vi "datatocsv.vi"(10 "FIT RESULTS":T1(array[cluster]), 11 "fit result data":cluster{"all rows":dbl[], "all rows":dbl[]}[](array[cluster])) -> (3 "error out":errorcluster)   [LabVIEW 2020]
uses:
  <vilib>/Utility/sysdir.llb/System Directory Type.ctl
panel:
  out "peakdata":string
  out "pltot data string":string
  out "path":path
  out "Array":dbl[][](array[numeric])
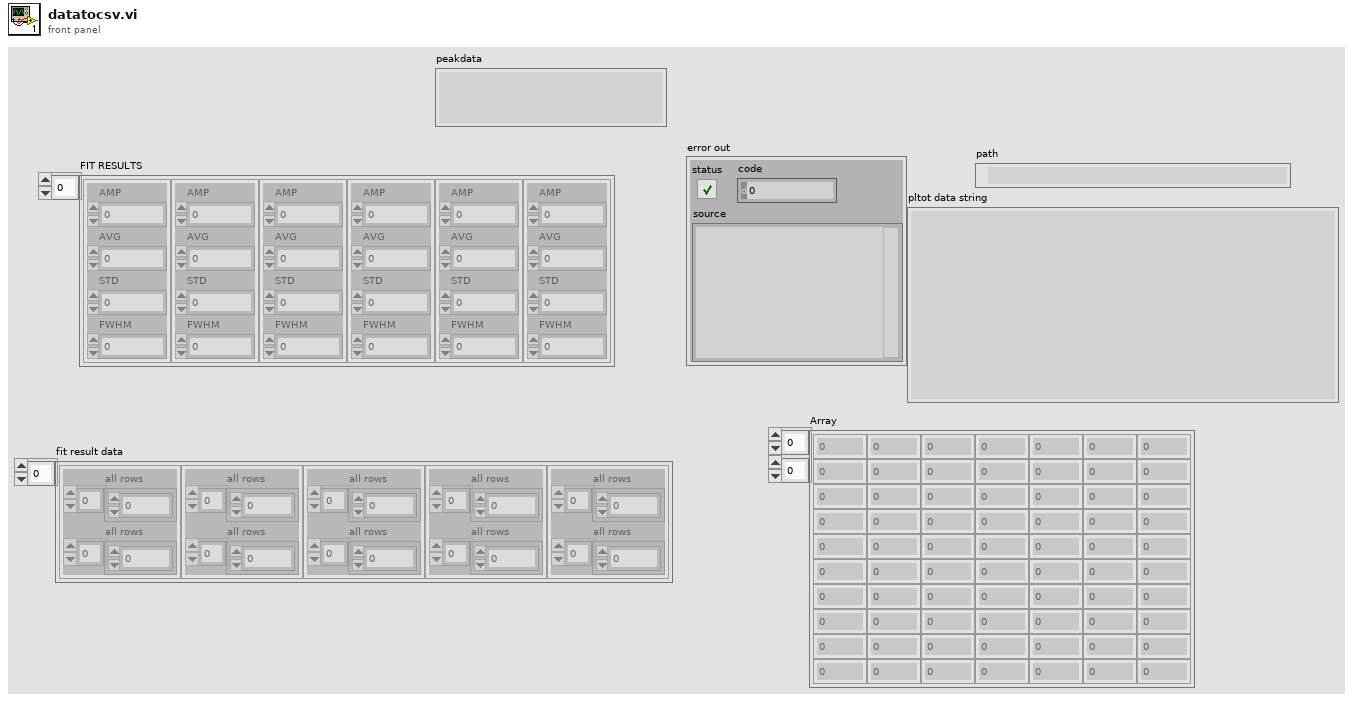
[diagram p1: front panel]
types:
  T1 = cluster{"AMP":dbl, "AVG":dbl, "STD":dbl, "FWHM":dbl}[]
  T2 = enum16{"open", "replace", "create", "open or create", "replace or create", "replace or create with confirmation"}
  T3 = typedef "System Directory Type.ctl" = i32
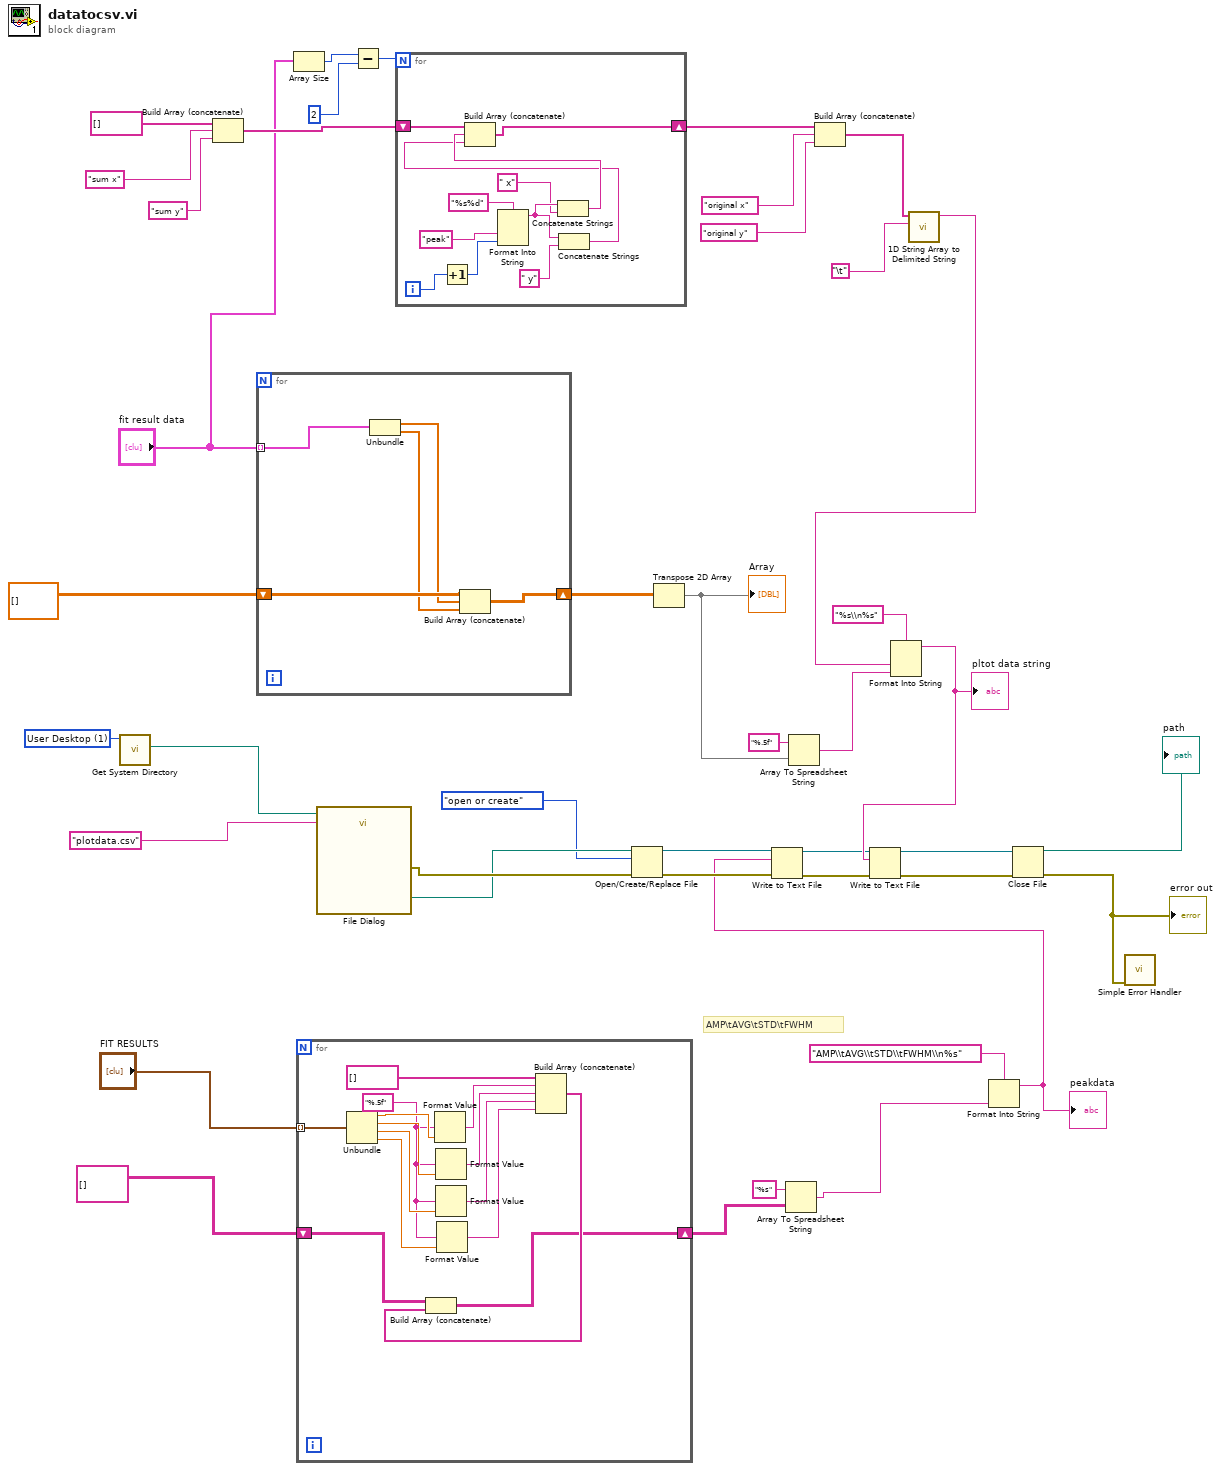
[diagram p0: block diagram]
diagram:
  w16 = T3 1 items=["User Home"=0, "User Desktop"=1, "User Documents"=2, "User Application Data"=3, "User Preferences"=4, "User Temporary"=5, "Public Documents"=6, "Public Application Data"=7, "Public Preferences"=8, "Public Cache"=13, "System Core Libraries"=9, "System Installed Libraries"=10, "Application Files"=11, "Boot Volume Root"=12] ("system directory type")
  # "AMP\\tAVG\\tSTD\\tFWHM"
  n1 = call <vilib>:"Get System Directory.vi"("system directory type"=w16) -> ("system directory"=w7:path)  [unwired: 10 in]
  n2 = Build Array (concatenate)(string[] [], "sum x", "sum y" ("element")) -> (w28:string[])
  n3 = for {
    tunnel: "fit result data" -> [w47] mode=indexing
    shift-right: [w43] -> w35
    shift-left: dbl[][] [] -> [w46]
    n4 = Unbundle(w47) -> ("all rows"=w45:dbl[], "all rows"=w44:dbl[])
    n5 = Build Array (concatenate)(w46, w45, w44) -> (w43:dbl[][])
  }
  n6 = Array Size(array="fit result data") -> (size(s)=w9:i32)
  n7 = for {
    tunnel: "FIT RESULTS" -> [w60] mode=indexing
    shift-right: [w57] -> w40
    shift-left: string[][] [] -> [w61]
    w48 = "%.5f" ("format string")
    n8 = Unbundle(w60) -> ("AMP"=w56:dbl, "AVG"=w55:dbl, "STD"=w54:dbl, "FWHM"=w53:dbl)
    n9 = Format Value(format string=w48, value (0)=w56) -> (output string=w52:string)  [unwired: 1 in]
    n10 = Format Value(format string=w48, value (0)=w55) -> (output string=w51:string)  [unwired: 1 in]
    n11 = Format Value(format string=w48, value (0)=w54) -> (output string=w50:string)  [unwired: 1 in]
    n12 = Format Value(format string=w48, value (0)=w53) -> (output string=w49:string)  [unwired: 1 in]
    n13 = Build Array (concatenate)(string[] [], w52, w51, w50, w49) -> (w58:string[])
    n14 = Build Array (concatenate)(w61, w58) -> (w57:string[][])
  }
  n15 = call "File Dialog"("start path"=w7, "default name"="plotdata.csv") -> ("selected path"=w12:path, "error out"=w17:errorcluster)  [unwired: 10 in, 2 out]
  n16 = Subtract(x=w9, y=2) -> (x-y=w27:i32)
  n17 = for {
    N: w27 -> [_]
    shift-right: [w67] -> w26
    shift-left: w28 -> [w71]
    i -> [w72]
    n18 = Increment(x=w72) -> (x+1=w68:i32)
    n19 = Format Into String(format string="%s%d", "peak", w68) -> (resulting string=w66:string)  [unwired: 2 in, 1 out]
    n20 = Concatenate Strings(w66, " x" ("string")) -> (w63:string)
    n21 = Concatenate Strings(w66, " y" ("string")) -> (w62:string)
    n22 = Build Array (concatenate)(w71, w63, w62) -> (w67:string[])
  }
  n23 = Open/Create/Replace File(file path (use dialog)=w12, error in=w17, operation (0:open)=T2."open or create") -> (refnum out=w5:refnum<file>, error out=w4:errorcluster)  [unwired: 3 in, 1 out]
  n24 = Transpose 2D Array(2D array=w35) -> (transposed array=w34:dbl[][])
  "Array" <- w34
  n25 = Array To Spreadsheet String(array=w40, 3:"%s" ("format string")) -> (spreadsheet string=w37:string)  [unwired: 1 in]
  n26 = Array To Spreadsheet String(array=w34, 3:"%.5f" ("format string")) -> (spreadsheet string=w32:string)  [unwired: 1 in]
  n27 = Build Array (concatenate)(w26, "original x", "original y") -> (w22:string[])
  n28 = call <vilib>:"1D String Array to Delimited String.vi"("delimiter"="\t", "string array"=w22) -> ("delimited string"=w20:string)  [unwired: 9 in]
  n29 = Format Into String(format string="%s\\n%s", w20, w32) -> (resulting string=w6:string)  [unwired: 2 in, 1 out]
  "pltot data string" <- w6
  n30 = Format Into String(format string="AMP\\tAVG\\tSTD\\tFWHM\\n%s", w37) -> (resulting string=w1:string)  [unwired: 2 in, 1 out]
  "peakdata" <- w1
  n31 = Write to Text File(file (use dialog)=w5, text=w1, error in=w4) -> (refnum out=w3:refnum<file>, error out=w2:errorcluster)  [unwired: 1 in, 1 out]
  n32 = Write to Text File(file (use dialog)=w3, text=w6, error in=w2) -> (refnum out=w19:refnum<file>, error out=w18:errorcluster)  [unwired: 1 in, 1 out]
  n33 = Close File(refnum=w19, error in=w18) -> (path=→"path":path, error out=w13:errorcluster)
  "error out" <- w13
  n34 = call <vilib>:"Simple Error Handler.vi"("error in (no error)"=w13) -> ()  [unwired: 4 in, 5 out]
